vi "Main.vi"() -> ()   [LabVIEW 2020]
uses:
  ControllerStates.ctl
  MoveFiles/Controller/TypeDefs/DataCluster.ctl
  CheckFileCorrectness/TypeDefs/DataCluster.ctl
  CheckFileCorrectness/CheckMeasurementCorrectness.lvlib
  MoveFiles/Controller/MoveFiles.lvlib
panel:
  out "Table Control":string[][](table)
  out "Injection Issue!":bool
  in  "Averaging - Rough/Medium/Smooth":i32(slide)=4 scale=3.0..5.0
  out "FileToMove":path
  out "ShouldMove?":bool
  in  "Maunal Move":bool
  in  "START":bool
  in  "QUIT":bool
  out "error IO":errorcluster
  # "Moving and Real Time Analysis\n1. Choose Source folder with data\n2. Choose Destination folder for moving\n3. Press Start\n\nProgram automatically detects RawData files and starts the Real-Time Analysis\nFor last measurement file - you can Force Move and analysis will be also done."
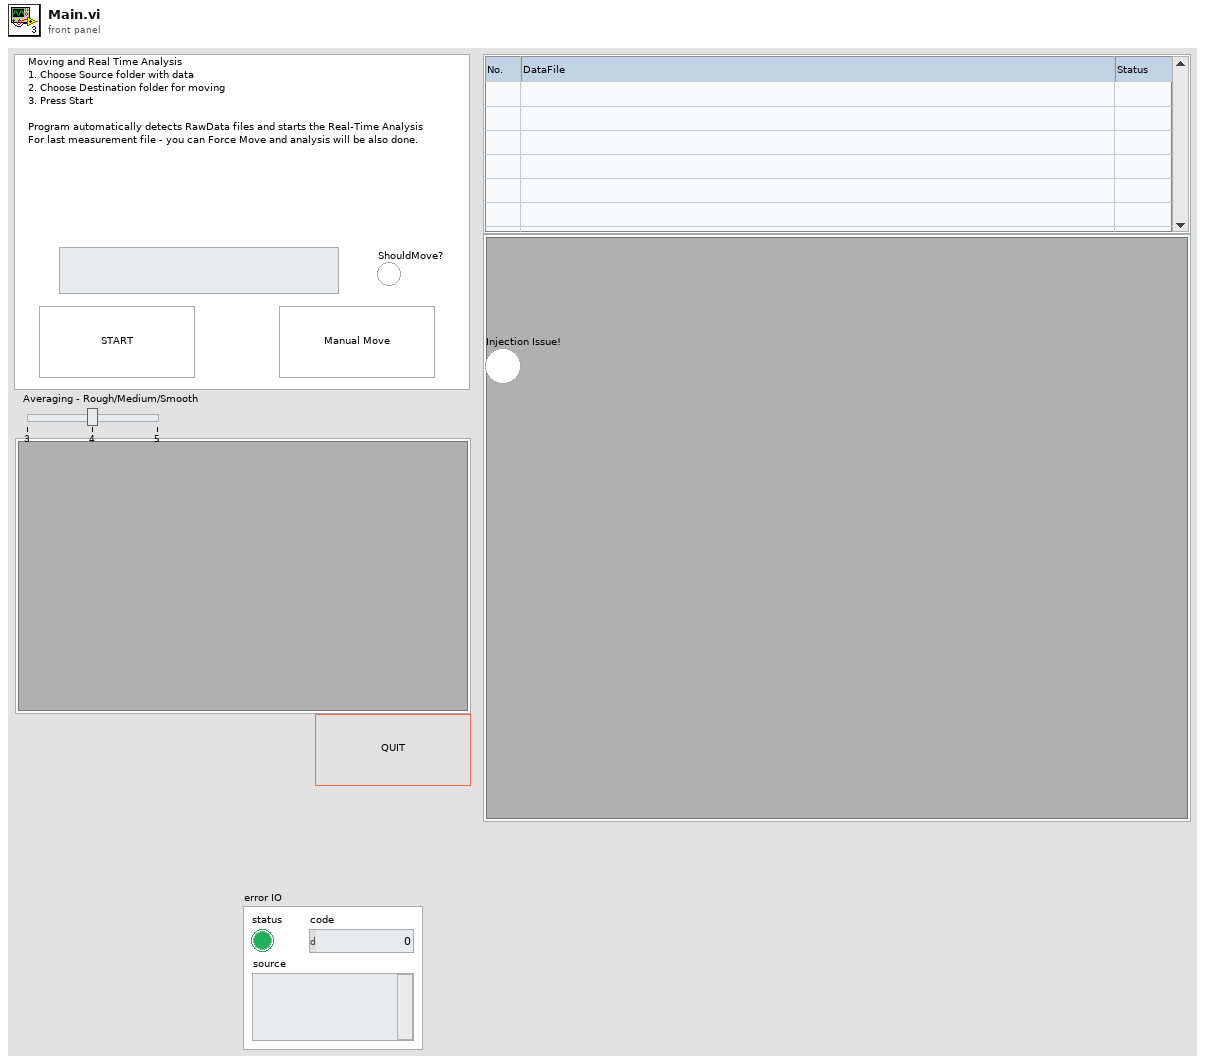
[diagram p1: front panel]
types:
  T1 = typedef "CheckMeasurementCorrectness.lvlib/DataCluster.ctl" = cluster{"File Path":path, "Type of Acquisition":enum16{"Single", "Dual", "Quad"}, "Averaging - Rough/Medium/Smooth":i32, "Finished?":bool, "Injection Issue!":bool}
  T2 = typedef "MoveFiles.lvlib/DataCluster.ctl" = cluster{"Fast Folder":path, "Slow Folder":path, "ShouldMove?":bool, "FileToMove":path, "MoveInProgress?":bool}
  T3 = typedef "ControllerStates.ctl" = enum16{"WaitingState", "GetDataForMoving", "ReadyForAnalysis?", "DoAnalysis", "IsFileAnalyzed?", "AllowMoving", "IsFileMoved?", "IgnoreIssue", "InjectionIssue", "ManualMove"}
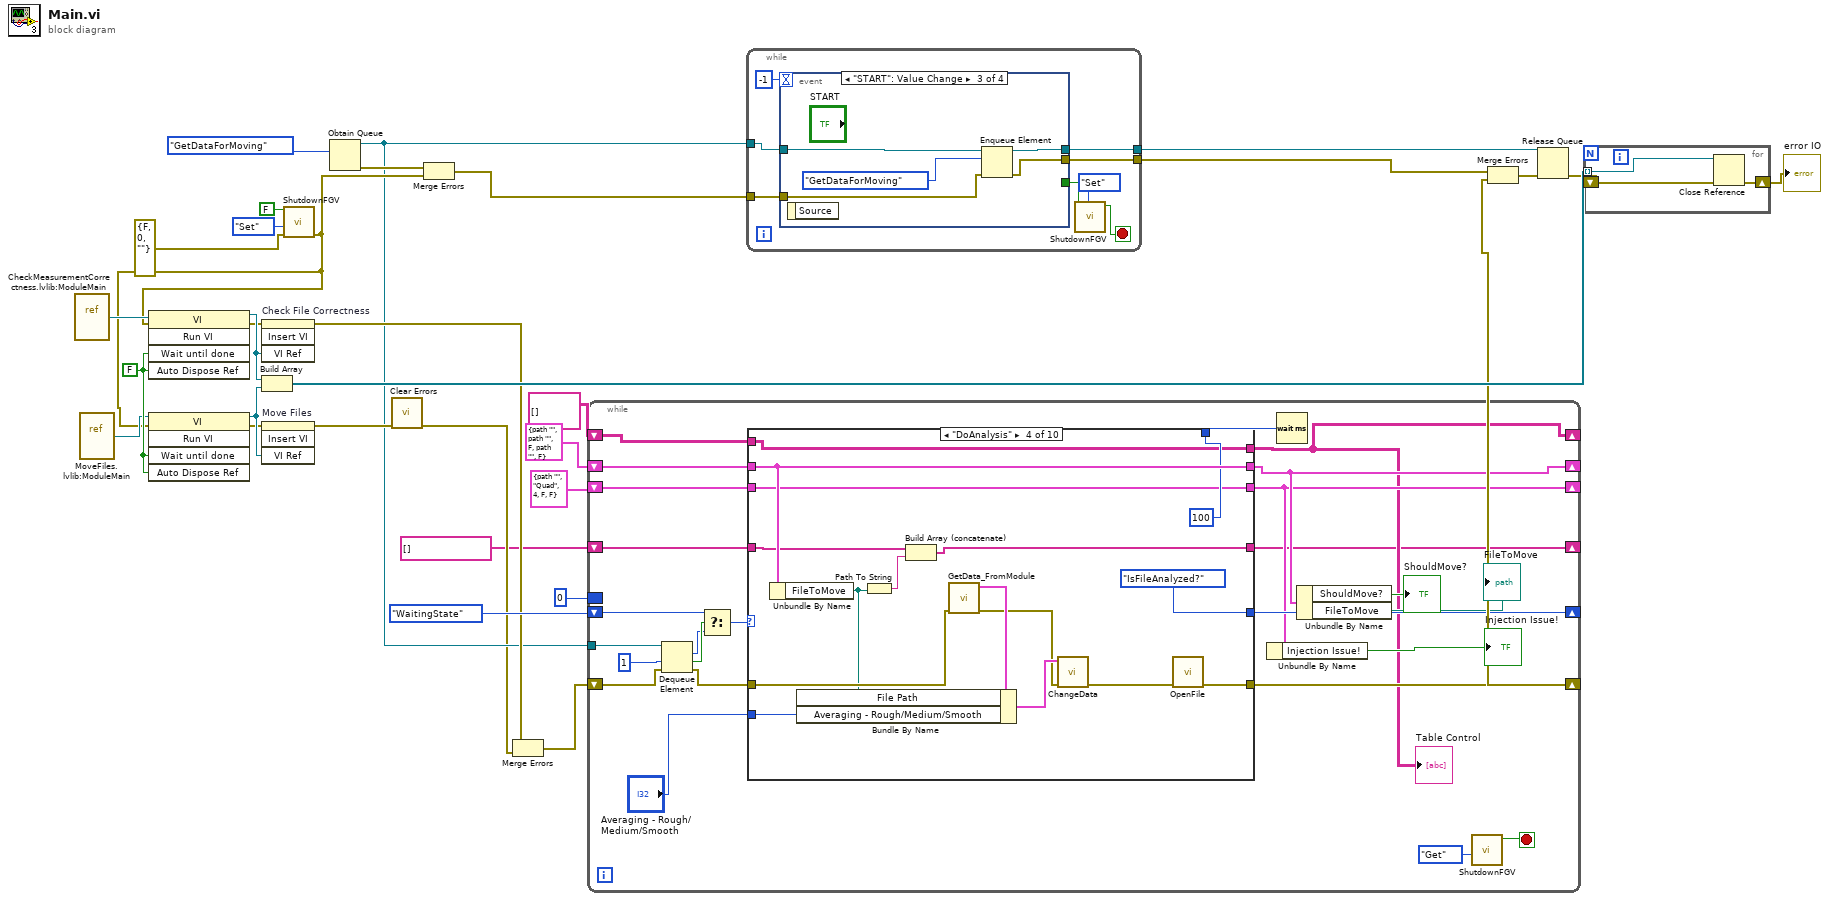
[diagram p0: block diagram]
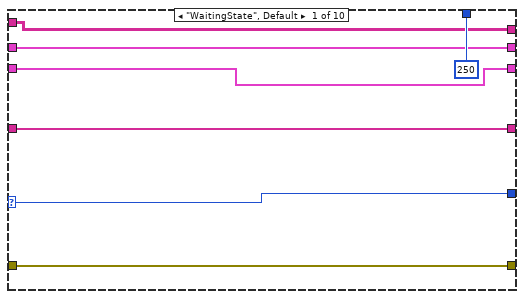
[diagram p2: hidden frame]
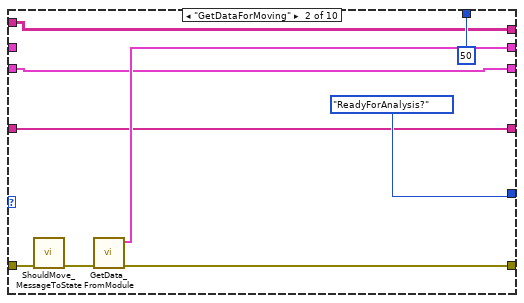
[diagram p3: hidden frame]
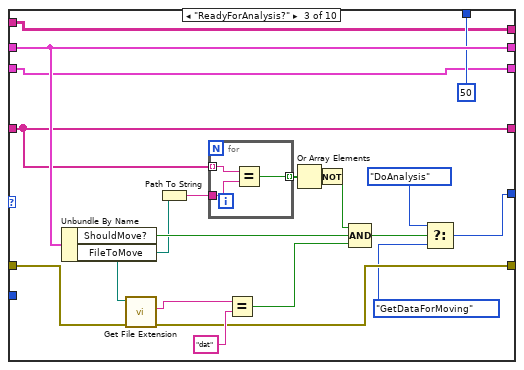
[diagram p4: hidden frame]
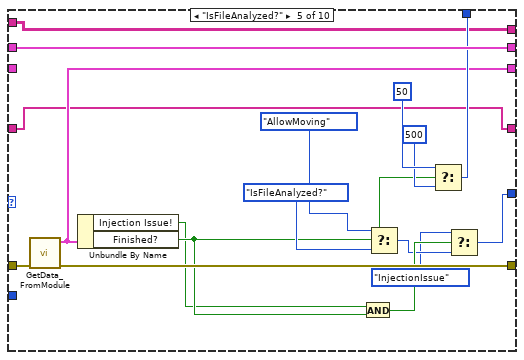
[diagram p5: hidden frame]
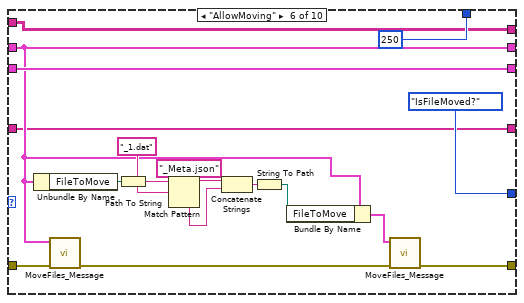
[diagram p6: hidden frame]
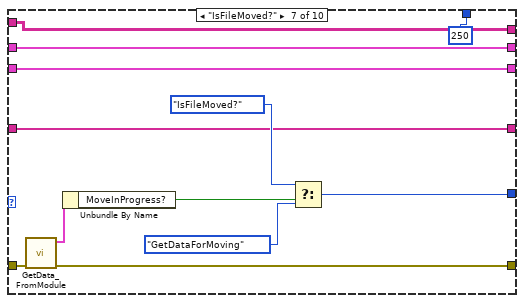
[diagram p7: hidden frame]
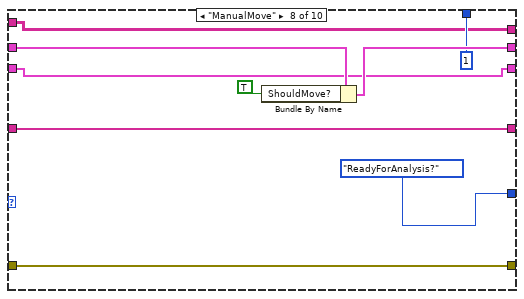
[diagram p8: hidden frame]
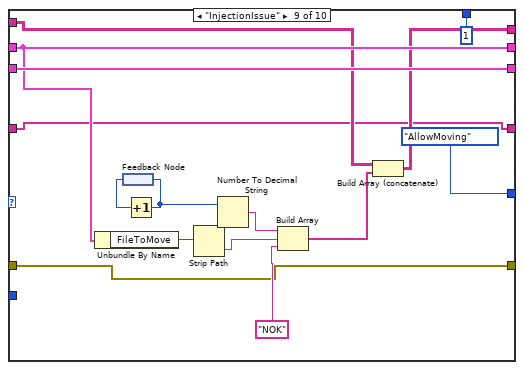
[diagram p9: hidden frame]
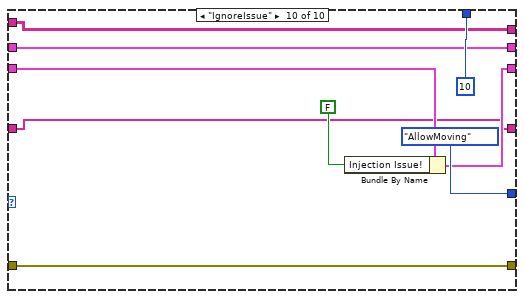
[diagram p10: hidden frame]
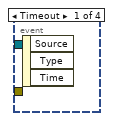
[diagram p11: hidden frame]
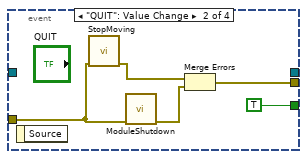
[diagram p12: hidden frame]
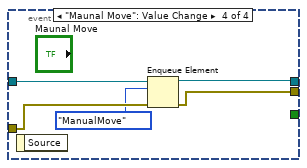
[diagram p13: hidden frame]
diagram:
  w32 = FALSE ("Wait Until Done")
  n1 = vi-ref "CheckMeasurementCorrectness.lvlib:ModuleMain.vi"() -> (w27:refnum<vi>)
  n2 = vi-ref "MoveFiles.lvlib:ModuleMain.vi"() -> (w26:refnum<vi>)
  n3 = call "ShutdownFGV.vi"("error in (no error)"=errorcluster {"status"=FALSE, "code"=0, "source"=""}, "Enum"=enum16{"Set", "Get"}."Set", "stop"=FALSE) -> ("error in (no error) 2"=w12:errorcluster)  [unwired: 7 in, 1 out]
  n4 = invoke class="VI" method="Run VI"(reference=w27, error in=w12, "Wait until done"=w32, "Auto Dispose Ref"=w32) -> (reference out=w28:refnum<vi>, error out=w18:errorcluster)  [unwired: 1 in, 3 out]
  n5 = invoke class="VI" method="Run VI"(reference=w26, error in=w12, "Wait until done"=w32, "Auto Dispose Ref"=w32) -> (reference out=w29:refnum<vi>, error out=w21:errorcluster)  [unwired: 1 in, 3 out]
  n6 = invoke on="Check File Correctness" class="SubPnl" method="Insert VI"(error in=w18, "VI Ref"=w28) -> (error out=w16:errorcluster)  [unwired: 2 in, 3 out]
  n7 = Build Array(w28, w29) -> (w30:refnum<vi>[])
  n8 = invoke on="Move Files" class="SubPnl" method="Insert VI"(error in=w21, "VI Ref"=w29) -> (error out=w15:errorcluster)  [unwired: 2 in, 3 out]
  n9 = Obtain Queue(element data type=ControllerStates."GetDataForMoving") -> (queue out=w10:refnum<queue>, error out=w13:errorcluster)  [unwired: 4 in, 1 out]
  n10 = call <vilib>:"Clear Errors.vi"("error in (no error)"=w15) -> ("error out"=w2:errorcluster)  [unwired: 5 in, 1 out]
  n11 = Merge Errors(w13, w12) -> (w11:errorcluster)
  n12 = Merge Errors(w16, w2) -> (w20:errorcluster)
  n13 = while {
    shift-right: [w55] -> w19
    shift-left: w20 -> [w49]
    shift-right: [w54] -> _
    shift-left: ControllerStates."WaitingState" -> [w45]
    shift-right: [w43] -> _
    shift-left: T2 {"Fast Folder"=path "", "Slow Folder"=path "", "ShouldMove?"=FALSE, "FileToMove"=path "", "MoveInProgress?"=FALSE} ("Data Out") -> [w53]
    tunnel: w10 -> [w51]
    shift-right: [w38] -> _
    shift-left: T1 {"File Path"=path "", "Type of Acquisition"=enum."Quad", "Averaging - Rough/Medium/Smooth"=4, "Finished?"=FALSE, "Injection Issue!"=FALSE} ("Data Out") -> [w39]
    shift-right: [w35] -> _
    shift-left: string[][] [] ("Table Control") -> [w36]
    border: 0 -> [_]
    shift-right: [w33] -> _
    shift-left: string[] [] -> [w34]
    stop <- w56 stop-if-true
    n14 = Dequeue Element(queue=w51, timeout in ms (-1)=1, error in (no error)=w49) -> (element=w46:T3, timed out?=w47:bool, error out=w48:errorcluster)  [unwired: 1 out]
    n15 = Select(t=w45, s=w47, f=w46) -> (s? t:f=w44:T3)
    n16 = case shown="\"DoAnalysis\"" w44 {
      selector: w44 -> [w64 _ _ _ _ _ _ _ _ _]
      tunnel: [w61 w69 w86 w110 w122 w131 w148 w162 w171 w187] -> w55
      tunnel: w48 -> [w61 w71 w89 w104 w129 w146 w149 w162 w171 w187]
      tunnel: [w64 ControllerStates."ReadyForAnalysis?" ("f") w87 ControllerStates."IsFileAnalyzed?" ("f") w116 ControllerStates."IsFileMoved?" ("f") w152 ControllerStates."ReadyForAnalysis?" ("f") ControllerStates."AllowMoving" ("f") ControllerStates."AllowMoving" ("f")] -> w54
      tunnel: [w62 w73 w88 w107 w128 w135 w156 w164 w178 w185] -> w43
      tunnel: w53 -> [w62 _ w88 w107 w128 w135 w156 w166 w178 w185]
      tunnel: [u32 250 ("f") u32 50 ("milliseconds to wait") u32 50 ("f") u32 100 ("milliseconds to wait") w124 u32 250 ("f") u32 250 ("f") u32 1 ("f") u32 1 ("f") u32 10 ("f")] -> w52
      tunnel: "Averaging - Rough/Medium/Smooth" -> [_ _ _ w103 _ _ _ _ _ _]
      tunnel: [w60 w67 w84 w102 w121 w143 w158 w161 w182 w186] -> w38
      tunnel: w39 -> [w60 w67 w84 w102 _ w143 w158 w161 w182 w189]
      tunnel: w36 -> [w59 w66 w83 w101 w114 w142 w157 w160 w177 w184]
      tunnel: [w59 w66 w83 w101 w114 w142 w157 w160 w176 w184] -> w35
      tunnel: w34 -> [w58 w65 w79 w100 w113 w130 w147 w159 w168 w183]
      tunnel: [w58 w65 w79 w97 w113 w130 w147 w159 w168 w183] -> w33
      frame "WaitingState", Default {
      }
      frame "GetDataForMoving" {
        n17 = call "ShouldMove_MessageToState.vi"("error in"=w71) -> ("error out"=w70:errorcluster)  [unwired: 10 in]
        n18 = call "GetData_FromModule.vi"("error in (no error)"=w70) -> ("error out"=w69:errorcluster, "Data Out"=w73:T2)  [unwired: 9 in]
      }
      frame "ReadyForAnalysis?" {
        n19 = Unbundle By Name(w88) -> ("ShouldMove?"=w92:bool, "FileToMove"=w78:path)
        n20 = call <vilib>:"Get File Extension.vi"("error in (no error)"=w89, "file"=w78) -> ("error out"=w86:errorcluster, "lowercase file extension"=w81:string)  [unwired: 5 in, 3 out]
        n21 = Path To String(path=w78) -> (string=w77:string)
        n22 = for {
          tunnel: w79 -> [w96] mode=indexing
          tunnel: w77 -> [w95]
          tunnel: [w94] -> w76 mode=indexing
          n23 = Equal?(x=w96, y=w95) -> (x = y?=w94:bool)
        }
        n24 = Equal?(x=w81, y="dat" ("x")) -> (x = y?=w82:bool)
        n25 = Or Array Elements(Boolean array=w76) -> (logical OR=w75:bool)
        n26 = Not(x=w75) -> (.not. x?=w74:bool)
        n27 = Compound Arithmetic op=AND(w74, w92, w82) -> (w91:bool)
        n28 = Select(t=ControllerStates."DoAnalysis", s=w91, f=ControllerStates."GetDataForMoving") -> (s? t:f=w87:T3)
      }
      frame "DoAnalysis" {
        n29 = Unbundle By Name(w107) -> ("FileToMove"=w99:path)
        n30 = Path To String(path=w99) -> (string=w98:string)
        n31 = Build Array (concatenate)(w100, w98) -> (w97:string[])
        n32 = call "GetData_FromModule.vi"("error in (no error)"=w104) -> ("error out"=w108:errorcluster, "Data Out"=w109:T1)  [unwired: 9 in]
        n33 = Bundle By Name(cluster=w109, "File Path"=w99, "Averaging - Rough/Medium/Smooth"=w103) -> (w112:T1)
        n34 = call "ChangeData.vi"("error in"=w108, "Cluster"=w112) -> ("error out"=w111:errorcluster)  [unwired: 9 in]
        n35 = call "OpenFile.vi"("error in"=w111) -> ("error out"=w110:errorcluster)  [unwired: 10 in]
      }
      frame "IsFileAnalyzed?" {
        n36 = call "GetData_FromModule.vi"("error in (no error)"=w129) -> ("error out"=w122:errorcluster, "Data Out"=w121:T1)  [unwired: 9 in]
        n37 = Unbundle By Name(w121) -> ("Injection Issue!"=w119:bool, "Finished?"=w120:bool)
        n38 = And(x=w119, y=w120) -> (x .and. y?=w118:bool)
        n39 = Select(t=ControllerStates."AllowMoving" ("f"), s=w120, f=ControllerStates."IsFileAnalyzed?") -> (s? t:f=w117:T3)
        n40 = Select(t=u32 50 ("milliseconds to wait"), s=w120, f=u32 500) -> (s? t:f=w124:u32)
        n41 = Select(t=ControllerStates."InjectionIssue", s=w118, f=w117) -> (s? t:f=w116:T3)
      }
      frame "AllowMoving" {
        n42 = Unbundle By Name(w135) -> ("FileToMove"=w140:path)
        n43 = call "MoveFiles_Message.vi"("error in"=w146, "DataToMove"=w135) -> ("error out"=w132:errorcluster)  [unwired: 9 in]
        n44 = Path To String(path=w140) -> (string=w139:string)
        n45 = Match Pattern(string=w139, regular expression="_1.dat") -> (before substring=w138:string)  [unwired: 1 in, 3 out]
        n46 = Concatenate Strings(w138, "_Meta.json" ("string")) -> (w136:string)
        n47 = String To Path(string=w136) -> (path=w134:path)
        n48 = Bundle By Name(cluster=w135, "FileToMove"=w134) -> (w133:T2)
        n49 = call "MoveFiles_Message.vi"("error in"=w132, "DataToMove"=w133) -> ("error out"=w131:errorcluster)  [unwired: 9 in]
      }
      frame "IsFileMoved?" {
        n50 = call "GetData_FromModule.vi"("error in (no error)"=w149) -> ("error out"=w148:errorcluster, "Data Out"=w150:T2)  [unwired: 9 in]
        n51 = Unbundle By Name(w150) -> ("MoveInProgress?"=w155:bool)
        n52 = Select(t=ControllerStates."IsFileMoved?", s=w155, f=ControllerStates."GetDataForMoving") -> (s? t:f=w152:T3)
      }
      frame "ManualMove" {
        n53 = Bundle By Name(cluster=w166, "ShouldMove?"=TRUE) -> (w164:T2)
      }
      frame "InjectionIssue" {
        n54 = Unbundle By Name(w178) -> ("FileToMove"=w170:path)
        n55 = feedback #1() -> (w181:i32)
        n56 = Increment(x=w181) -> (x+1=w180:i32)
        n57 = feedback-in #1(w180) -> ()
        n58 = Strip Path(path=w170) -> (name=w169:string)  [unwired: 1 out]
        n59 = Number To Decimal String(number=w180) -> (decimal integer string=w179:string)  [unwired: 1 in]
        n60 = Build Array(w179, w169, "NOK" ("element")) -> (w174:string[])
        n61 = Build Array (concatenate)(w177, w174) -> (w176:string[][])
      }
      frame "IgnoreIssue" {
        n62 = Bundle By Name(cluster=w189, "Injection Issue!"=FALSE) -> (w186:T1)
      }
    }
    "Table Control" <- w35
    n63 = Unbundle By Name(w38) -> ("Injection Issue!"=→"Injection Issue!":bool)
    n64 = Wait (ms)(milliseconds to wait=w52) -> ()  [unwired: 1 out]
    n65 = Unbundle By Name(w43) -> ("ShouldMove?"=→"ShouldMove?":bool, "FileToMove"=→"FileToMove":path)
    n66 = call "ShutdownFGV.vi"("Enum"=enum16{"Set", "Get"}."Get") -> ("Boolean"=w56:bool)  [unwired: 9 in, 1 out]
  }
  n67 = while {
    tunnel: w11 -> [w199]
    tunnel: [w198] -> w7
    tunnel: w10 -> [w193]
    tunnel: [w192] -> w8
    stop <- w195 stop-if-true
    n68 = event shown="[2] \"START\": Value Change" {
      selector: _ -> [_ _ _ _]
      dyn-events: _ -> [_ _ _ _]
      timeout: -1 -> [_ _ _ _]
      tunnel: [_ TRUE _ _] -> w196
      tunnel: w199 -> [_ w203 w206 w212]
      tunnel: [_ w201 w205 w210] -> w198
      tunnel: w193 -> [_ _ w209 w214]
      tunnel: [_ _ w208 w213] -> w192
      event Timeout {
        n69 = event-data() -> ()  [unwired: 1 in, 3 out]
      }
      event "QUIT": Value Change {
        n70 = event-data() -> ()  [unwired: 1 in, 1 out]
        n71 = call "StopMoving.vi"("error in"=w203) -> ("error out"=w200:errorcluster)  [unwired: 10 in]
        n72 = call "ModuleShutdown.vi"("error in"=w203) -> ("error out"=w202:errorcluster)  [unwired: 10 in]
        n73 = Merge Errors(w200, w202) -> (w201:errorcluster)
      }
      event "START": Value Change {
        n74 = event-data() -> ()  [unwired: 1 in, 1 out]
        n75 = Enqueue Element(queue=w209, element=ControllerStates."GetDataForMoving", error in (no error)=w206) -> (queue out=w208:refnum<queue>, error out=w205:errorcluster)  [unwired: 1 in, 1 out]
      }
      event "Maunal Move": Value Change {
        n76 = event-data() -> ()  [unwired: 1 in, 1 out]
        n77 = Enqueue Element(queue=w214, element=ControllerStates."ManualMove", error in (no error)=w212) -> (queue out=w213:refnum<queue>, error out=w210:errorcluster)  [unwired: 1 in, 1 out]
      }
    }
    n78 = call "ShutdownFGV.vi"("Enum"=enum16{"Set", "Get"}."Set", "stop"=w196) -> ("Boolean"=w195:bool)  [unwired: 8 in, 1 out]
  }
  n79 = Merge Errors(w7, w19) -> (w31:errorcluster)
  n80 = Release Queue(queue=w8, error in (no error)=w31) -> (error out=w9:errorcluster)  [unwired: 1 in, 2 out]
  n81 = for {
    shift-right: [w216] -> w25
    shift-left: w9 -> [w217]
    tunnel: w30 -> [w215] mode=indexing
    n82 = Close Reference(reference=w215, error in (no error)=w217) -> (error out=w216:errorcluster)
  }
  "error IO" <- w25
